vi "Enqueue Message and Wait for Response.vi"(4 "timeout in ms (-1)":i32=-1, 6 "priority message (T)":bool=TRUE, 8 "error in":errorcluster, 9 "message data":variant, 10 "message":string, 11 "message queue":refnum<queue>) -> (0 "error out":errorcluster, 1 "reply message data":variant, 2 "reply message":string, 3 "dup message queue":refnum<queue>)   [LabVIEW 2024, in "DSA_CFG_ACQ.lvlib" / "SFPMessage Queue.lvlib"]
doc: "For a regular message, enqueue the message. For a priority message, enqueue it at the front of the queue."
uses:
  SFPMessage Queue.lvlib
  Message Cluster.ctl
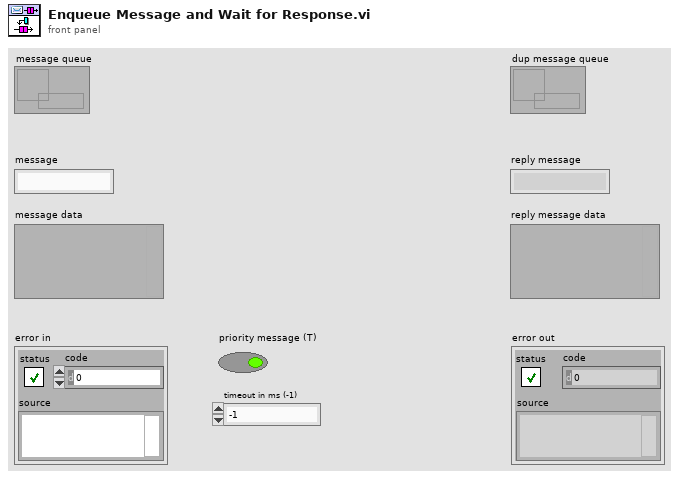
[diagram p1: front panel]
types:
  T1 = typedef "DSA_CFG_ACQ.lvlib/SFPMessage Queue.lvlib/Message Cluster.ctl" = cluster{"Message":string, "Message Data":variant}
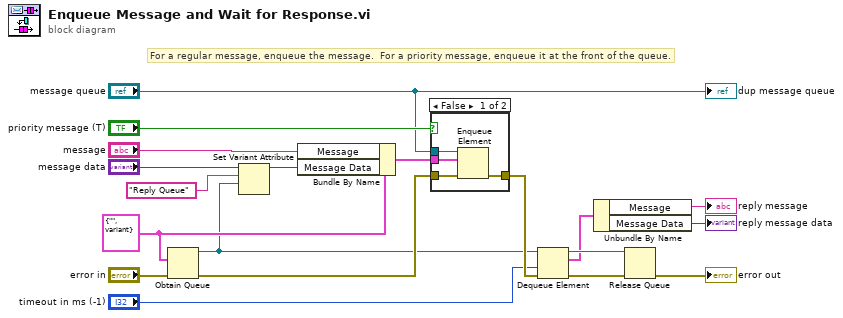
[diagram p0: block diagram]
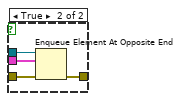
[diagram p2: hidden frame]
diagram:
  w8 = T1 {"Message"="", "Message Data"=variant} ("Message Cluster")
  # "For a regular message, enqueue the message.  For a priority message, enqueue it at the front of the queue."
  n1 = Obtain Queue(element data type=w8, error in (no error)="error in") -> (queue out=w5:refnum<queue>, error out=w10:errorcluster)  [unwired: 3 in, 1 out]
  n2 = Set Variant Attribute(Variant="message data", name="Reply Queue", value=w5) -> (Variant out=w6:variant)  [unwired: 1 in, 2 out]
  n3 = Bundle By Name(cluster=w8, "Message"="message", "Message Data"=w6) -> (w9:T1)
  n4 = case shown="False" "priority message (T)" {
    tunnel: w10 -> [w23 w27]
    tunnel: [w22 w26] -> w14
    tunnel: "message queue" -> [w21 w25]
    tunnel: w9 -> [w20 w24]
    frame False {
      n5 = Enqueue Element(queue=w21, element=w20, error in (no error)=w23) -> (error out=w22:errorcluster)  [unwired: 1 in, 2 out]
    }
    frame True {
      n6 = Enqueue Element At Opposite End(queue=w25, element=w24, error in (no error)=w27) -> (error out=w26:errorcluster)  [unwired: 1 in, 2 out]
    }
  }
  n7 = Dequeue Element(queue=w5, timeout in ms (-1)="timeout in ms (-1)", error in (no error)=w14) -> (queue out=w15:refnum<queue>, element=w3:T1, error out=w16:errorcluster)  [unwired: 1 out]
  n8 = Unbundle By Name(w3) -> ("Message"=→"reply message":string, "Message Data"=→"reply message data":variant)
  n9 = Release Queue(queue=w15, error in (no error)=w16) -> (error out=→"error out":errorcluster)  [unwired: 1 in, 2 out]
  "dup message queue" <- "message queue"
